vi "Update_VelocityProfileMove.vi"(6 "Skip Update?":bool, 8 "error in (no error)":errorcluster, 9 "StatusWord":u16, 10 "ControlWord":u16 format="%.0b", 11 "SoftmotionAxis in":refnum<class "SoftmotionAxis.lvclass">) -> (0 "error out":errorcluster, 1 "StatusWord Out":u16, 3 "SoftmotionAxis out":refnum<class "SoftmotionAxis.lvclass">)   [LabVIEW 2017, in "SoftmotionAxis.lvclass"]
uses:
  SoftmotionAxis.lvclass
  Utilities/Bit Manipulation.lvlib
  <resource>/objmgr/nimcai.rc
  <resource>/objmgr/nimotion.rc
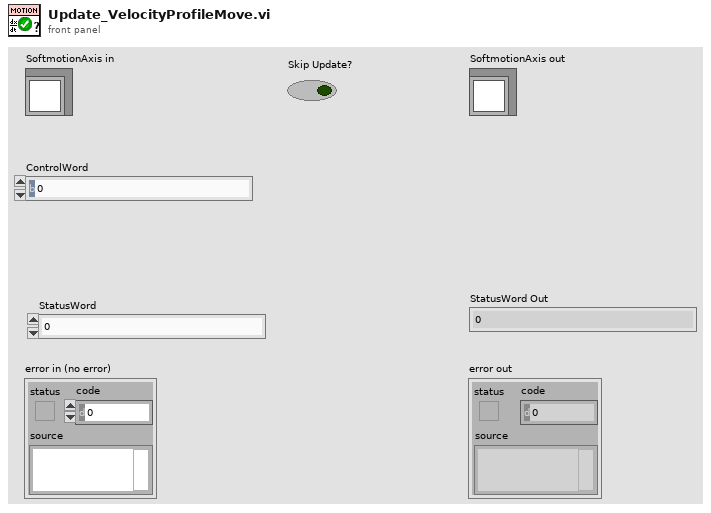
[diagram p1: front panel]
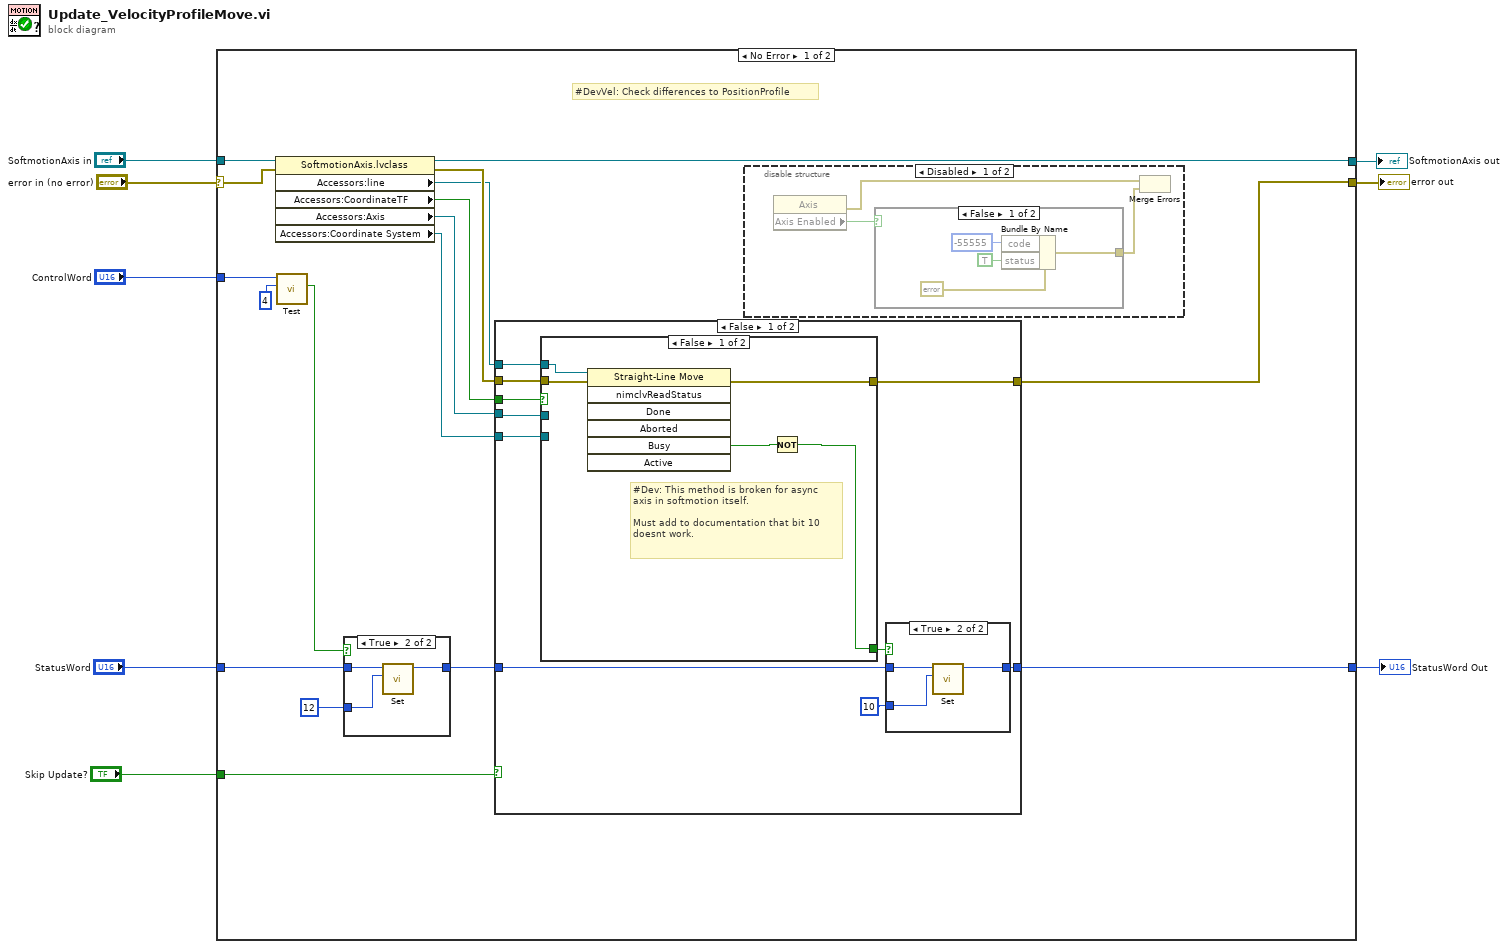
[diagram p0: block diagram]
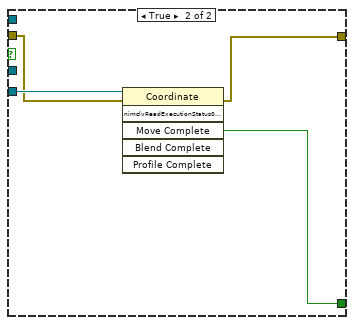
[diagram p4: hidden frame]
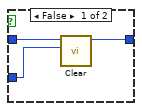
[diagram p5: hidden frame]
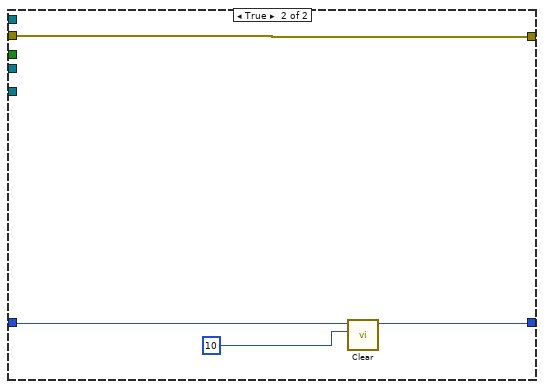
[diagram p6: hidden frame]
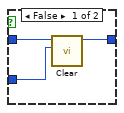
[diagram p7: hidden frame]
diagram:
  n1 = case shown="No Error" "error in (no error)" {
    selector: "error in (no error)" -> [w23 w70]
    tunnel: [w10 w70] -> w7
    tunnel: [w16 w69] -> w5
    tunnel: "SoftmotionAxis in" -> [w24 w69]
    tunnel: "StatusWord" -> [w22 w68]
    tunnel: [w25 w68] -> w3
    tunnel: "ControlWord" -> [w20 _]
    tunnel: "Skip Update?" -> [w15 _]
    frame No Error {
      # "#DevVel: Check differences to PositionProfile"
      n2 = property class="SoftmotionAxis.lvclass"(reference=w24, error in=w23) -> (reference out=w16:refnum<class "SoftmotionAxis.lvclass">, error out=w11:errorcluster, "Accessors:line"=w9:refnum<k20>, "Accessors:CoordinateTF"=w14:bool, "Accessors:Axis"=w13:refnum<k21>, "Accessors:Coordinate System"=w12:refnum<k21>)
      n3 = call "Test.vi"("Bit to test"=u8 4, "Data_In"=w20) -> ("bit value"=w18:bool)  [unwired: 8 in, 1 out]
      n4 = case shown="True" w18 {
        tunnel: w22 -> [w64 w66]
        tunnel: [w63 w67] -> w21
        tunnel: u8 12 -> [w62 w65]
        frame False {
          n5 = call "Clear.vi"("Bit to clear"=w62, "Data_In"=w64) -> ("Data_Out"=w63:u16)  [unwired: 9 in]
        }
        frame True {
          n6 = call "Set.vi"("Bit to set"=w65, "Data_In"=w66) -> ("Data_Out"=w67:u16)  [unwired: 9 in]
        }
      }
      n7 = case shown="False" w15 {
        tunnel: [w41 w61] -> w25
        tunnel: w21 -> [w40 w60]
        tunnel: w13 -> [w39 _]
        tunnel: w14 -> [w37 _]
        tunnel: w12 -> [w36 _]
        tunnel: w11 -> [w35 w58]
        tunnel: [w34 w58] -> w10
        tunnel: w9 -> [w33 _]
        frame False {
          n8 = case shown="False" w37 {
            tunnel: w39 -> [_ _]
            tunnel: [w43 w50] -> w38
            tunnel: w36 -> [_ w51]
            tunnel: w35 -> [w46 w49]
            tunnel: [w45 w48] -> w34
            tunnel: w33 -> [w47 _]
            frame False {
              # "#Dev: This method is broken for async\naxis in softmotion itself. \n\nMust add to documentation that bit 10 \ndoesnt work."
              n9 = invoke class="Straight-Line Move" method="nimclvReadStatus"(reference=w47, error in=w46) -> (error out=w45:errorcluster, "Busy"=w44:bool)  [unwired: 5 in, 5 out]
              n10 = Not(x=w44) -> (.not. x?=w43:bool)
            }
            frame True {
              n11 = invoke class="Coordinate" method="nimclvReadExecutionStatus00A10011"(reference=w51, error in=w49) -> (error out=w48:errorcluster, "Move Complete"=w50:bool)  [unwired: 4 in, 4 out]
            }
          }
          n12 = case shown="True" w38 {
            tunnel: w40 -> [w54 w57]
            tunnel: [w53 w56] -> w41
            tunnel: u8 10 -> [w52 w55]
            frame False {
              n13 = call "Clear.vi"("Bit to clear"=w52, "Data_In"=w54) -> ("Data_Out"=w53:u16)  [unwired: 9 in]
            }
            frame True {
              n14 = call "Set.vi"("Bit to set"=w55, "Data_In"=w57) -> ("Data_Out"=w56:u16)  [unwired: 9 in]
            }
          }
        }
        frame True {
          n15 = call "Clear.vi"("Bit to clear"=u8 10, "Data_In"=w60) -> ("Data_Out"=w61:u16)  [unwired: 9 in]
        }
      }
      n16 = disable-structure shown="Disabled" {
        frame Disabled {
          n17 = property class="Axis"() -> (error out=w26:errorcluster, "Axis Enabled"=w28:bool)  [unwired: 2 in, 1 out]
          n18 = case shown="False" w28 {
            tunnel: [w29 _] -> w27
            frame False {
              n19 = Bundle By Name(cluster=errorcluster {"status"=FALSE, "code"=0, "source"=""} ("error in (no error)"), "code"=-55555, "status"=TRUE) -> (w29:errorcluster)
            }
            frame True {
            }
          }
          n20 = Merge Errors(w26, w27) -> ()  [unwired: 1 out]
        }
        frame Enabled {
        }
      }
    }
    frame Error {
    }
  }
  "error out" <- w7
  "SoftmotionAxis out" <- w5
  "StatusWord Out" <- w3
